vi "数据查询_数据查询.vi"() -> ()   [LabVIEW 2016]
uses:
  <vilib>/Utility/miscctls.llb/LVPointTypeDef.ctl
  <vilib>/Utility/miscctls.llb/LVRowAndColumnUnsignedTypeDef.ctl
  <vilib>/addons/database/_DB Variant To Data/Database Variant To Data.xnode
  SQL/database.lvlib
panel:
  out "连接的字符串":string
  out "选中数据表":string
  in  "查询":bool
  in  "结束日期":string="2020/01/01"
  in  "起始日期":string="2010/01/01"
  out "XY图":cluster{"data":timestamp[], "data":dbl[]}[](graph)
  in  "组合框":string(combo)
  out "数据表":string[][](table)
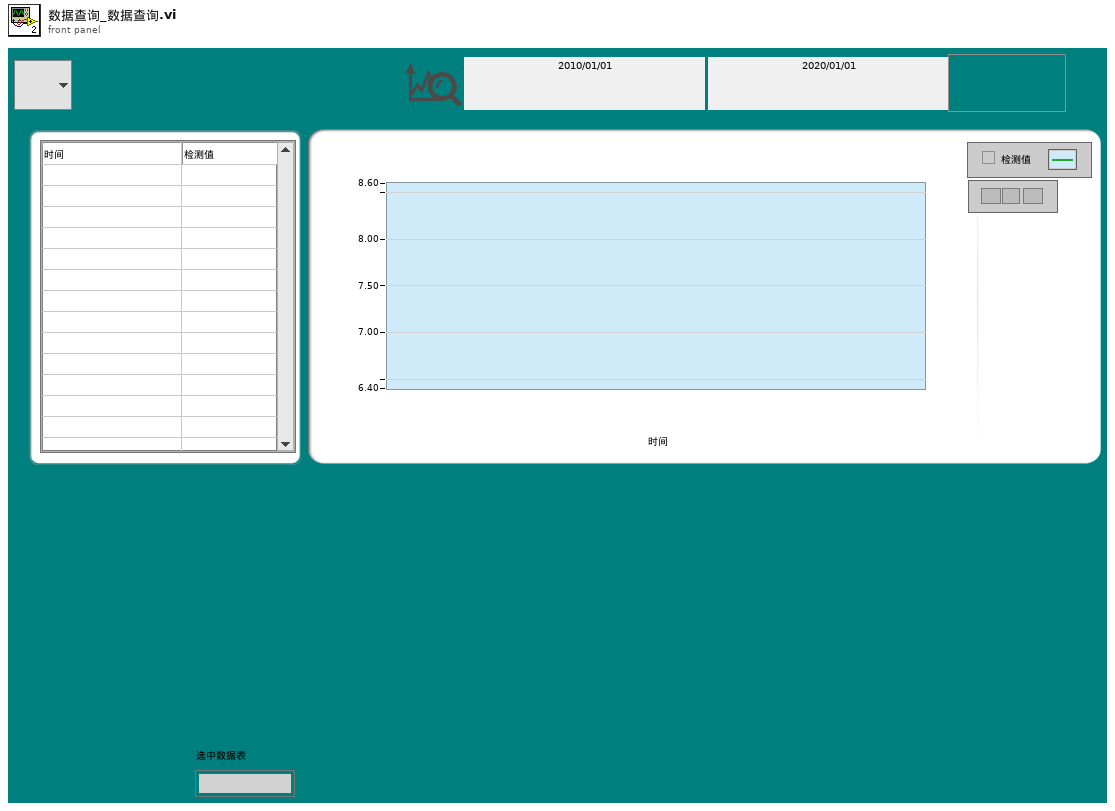
[diagram p1: front panel]
types:
  T1 = typedef "LVPointTypeDef.ctl" = cluster{"Horizontal":i16, "Vertical":i16}
  T2 = typedef "LVRowAndColumnUnsignedTypeDef.ctl" = cluster{"Row":u32, "Column":u32}
  T3 = typedef "LVPoint32TypeDef.ctl" = cluster{"Horizontal":i32, "Vertical":i32}
  T4 = typedef "LVPointDoubleTypeDef.ctl" = cluster{"Cursor X":dbl, "Cursor Y":dbl}
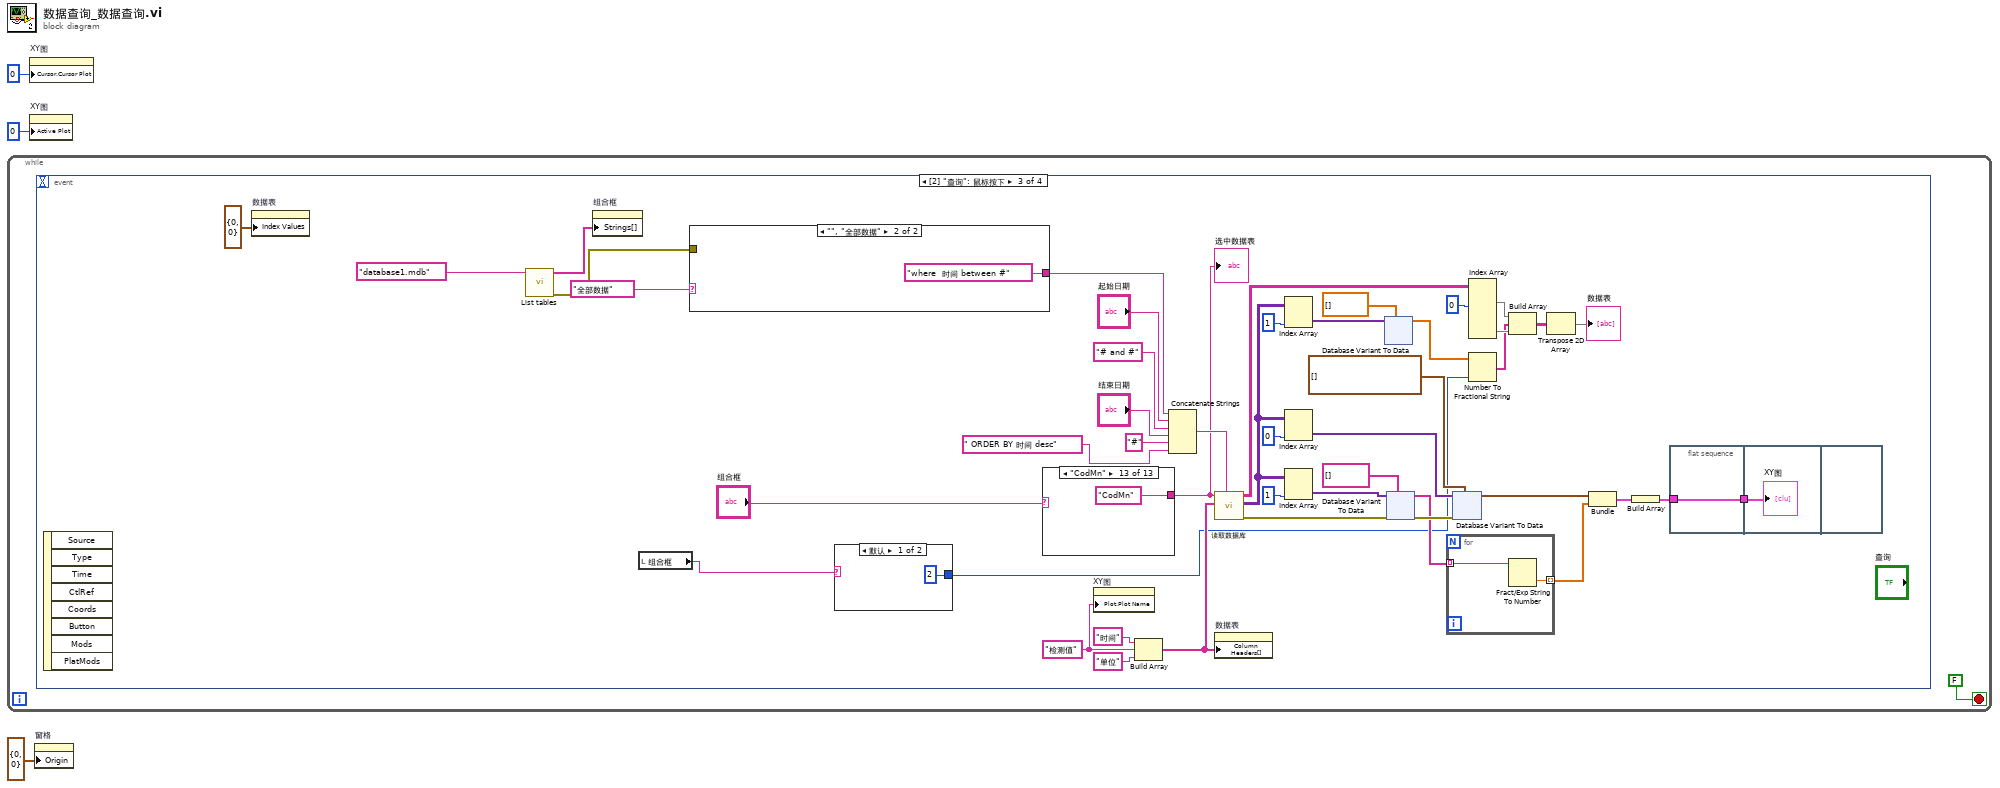
[diagram p0: block diagram]
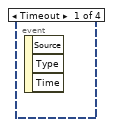
[diagram p2: hidden frame]
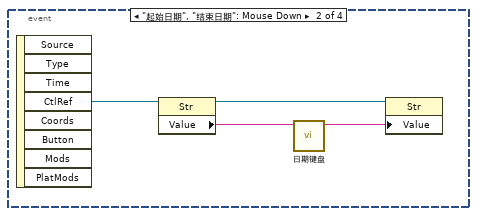
[diagram p3: hidden frame]
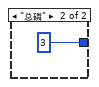
[diagram p4: hidden frame]
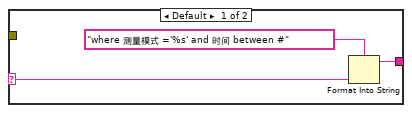
[diagram p5: hidden frame]
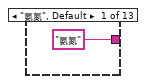
[diagram p6: hidden frame]
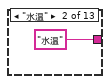
[diagram p7: hidden frame]
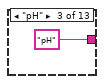
[diagram p8: hidden frame]
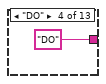
[diagram p9: hidden frame]
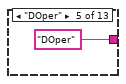
[diagram p10: hidden frame]
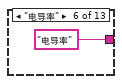
[diagram p11: hidden frame]
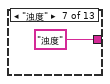
[diagram p12: hidden frame]
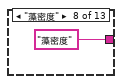
[diagram p13: hidden frame]
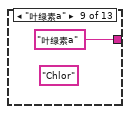
[diagram p14: hidden frame]
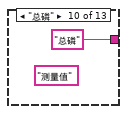
[diagram p15: hidden frame]
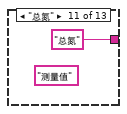
[diagram p16: hidden frame]
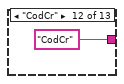
[diagram p17: hidden frame]
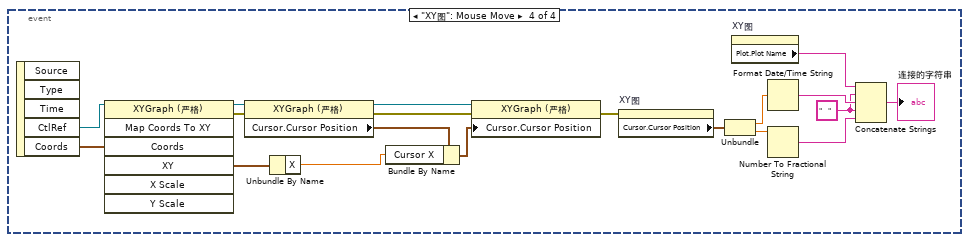
[diagram p18: hidden frame]
diagram:
  n1 = while {
    stop <- FALSE stop-if-true
    n2 = event shown="[2] \"查询\": 鼠标按下" {
      selector: _ -> [_ _ _ _]
      dyn-events: _ -> [_ _ _ _]
      timeout: _ -> [_ _ _ _]
      event Timeout {
        n3 = event-data() -> ()  [unwired: 1 in, 3 out]
      }
      event "起始日期", "结束日期": Mouse Down {
        n4 = event-data() -> ("CtlRef"=w8:refnum<vi>)  [unwired: 1 in, 7 out]
        n5 = property class="Str"(reference=w8) -> (reference out=w6:refnum<vi>, "Value"=w7:string)  [unwired: 1 in, 1 out]
        n6 = call "日期键盘.vi"("原值"=w7) -> ("x+y"=w5:string)  [unwired: 10 in]
        n7 = property class="Str"(reference=w6, "Value"=w5) -> ()  [unwired: 1 in, 2 out]
      }
      event "查询": Mouse Down {
        w26 = "检测值"
        n8 = event-data() -> ()  [unwired: 1 in, 8 out]
        n9 = property on="数据表" class="Tbl (严格)"("Index Values"=T2 {"Row"=0, "Column"=0} ("索引值")) -> ()  [unwired: 2 in, 2 out]
        n10 = call "List tables.vi"("database"="database1.mdb") -> ("error out"=w11:errorcluster, "tables"=w12:string[])  [unwired: 9 in]
        n11 = property on="组合框" class="CmbBox"("Strings[]"=w12) -> ()  [unwired: 2 in, 2 out]
        n12 = local read "组合框"() -> (w10:string)
        n13 = case shown="\"\", \"全部数据\"" "全部数据" ("工作模式") {
          selector: "全部数据" ("工作模式") -> [w59 _]
          tunnel: [w57 "where  时间 between #" ("condition")] -> w15
          tunnel: w11 -> [_ _]
          frame Default {
            n14 = Format Into String(format string="where 测量模式 ='%s' and 时间 between #" ("condition"), w59) -> (resulting string=w57:string)  [unwired: 2 in, 1 out]
          }
          frame "", "全部数据" {
          }
        }
        n15 = case shown="默认" w10 {
          tunnel: [i16 2 ("精度(6)") i16 3 ("精度(6)")] -> w9
          frame Default {
          }
          frame "总磷" {
          }
        }
        n16 = case shown="\"CodMn\"" "组合框" {
          tunnel: ["氨氮" "水温" "pH" "DO" "DOper" "电导率" "浊度" "藻密度" "叶绿素a" "总磷" "总氮" "CodCr" "CodMn"] -> w28
          frame "氨氮", Default {
          }
          frame "水温" {
          }
          frame "pH" {
          }
          frame "DO" {
          }
          frame "DOper" {
          }
          frame "电导率" {
          }
          frame "浊度" {
          }
          frame "藻密度" {
          }
          frame "叶绿素a" {
            (unwired) "Chlor"
          }
          frame "总磷" {
            (unwired) "测量值"
          }
          frame "总氮" {
            (unwired) "测量值"
          }
          frame "CodCr" {
          }
          frame "CodMn" {
          }
        }
        "选中数据表" <- w28
        n17 = property on="XY图" class="XYGraph (严格)"("Plot.Plot Name"=w26) -> ()  [unwired: 2 in, 2 out]
        n18 = Build Array("时间", w26, "单位" ("元素")) -> (w29:string[])
        n19 = Concatenate Strings(w15, "起始日期", "# and #" ("condition"), "结束日期", "#" ("condition"), " ORDER BY 时间 desc" ("字符串")) -> (w53:string)
        n20 = call "读取数据库.vi"("condition"=w53, "显示项"=w29, "组合框"=w28) -> ("error out"=w44:errorcluster, "data"=w23:variant[][], "表格"=w36:string[][])  [unwired: 5 in, 1 out]
        n21 = property on="数据表" class="Tbl (严格)"("Column Headers[]"=w29) -> ()  [unwired: 2 in, 2 out]
        n22 = Index Array(array=w23, index (col)=1 ("禁用的索引 (列)")) -> (element=w21:variant[])  [unwired: 1 in]
        n23 = Index Array(array=w23, index (col)=0 ("禁用的索引 (列)")) -> (element=w47:variant[])  [unwired: 1 in]
        n24 = Index Array(array=w23, index (col)=1 ("禁用的索引 (列)")) -> (element=w45:variant[])  [unwired: 1 in]
        n25 = xnode "Database Variant To Data"("database variant"=w21, "type"=sgl[] []) -> ("data"=w19:sgl[])  [unwired: 1 in, 1 out]
        n26 = xnode "Database Variant To Data"("database variant"=w45, "error in (no error)"=w44, "type"=string[] []) -> ("data"=w27:string[], "error out"=w43:errorcluster)
        n27 = for {
          tunnel: w27 -> [w100] mode=indexing
          tunnel: [w99] -> w14 mode=indexing
          n28 = Fract/Exp String To Number(string=w100) -> (number=w99:dbl)  [unwired: 3 in, 1 out]
        }
        n29 = xnode "Database Variant To Data"("database variant"=w47, "error in (no error)"=w43, "type"=timestamp[] []) -> ("data"=w38:timestamp[])  [unwired: 1 out]
        n30 = Index Array(array=w36, index (col) #1=0 ("禁用的索引 (列)")) -> (element #1=w34:string[], element #3=w24:string[])  [unwired: 5 in, 1 out]
        n31 = Number To Fractional String(number=w19, precision (6)=w9) -> (F-format string=w18:string[])  [unwired: 2 in]
        n32 = Build Array(w34, w18, w24) -> (w33:string[][])
        n33 = Transpose 2D Array(2D array=w33) -> (transposed array=→"数据表":string[][])
        n34 = Bundle("data"=w38, w14) -> (w39:cluster{"data":timestamp[], dbl[]})  [unwired: 1 in]
        n35 = Build Array(w39) -> (w40:cluster{"data":timestamp[], dbl[]}[])
        n36 = flat-sequence {
          tunnel: [w114] -> w41
          tunnel: w40 -> [w114]
          tunnel: w41 -> [w115]
          frame #0 {
          }
          frame #1 {
            "XY图" <- w115
          }
          frame #2 {
          }
        }
      }
      event "XY图": Mouse Move {
        w217 = "   " ("字符串")
        n37 = event-data() -> ("CtlRef"=w224:refnum<vi>, "Coords"=w223:T3)  [unwired: 1 in, 3 out]
        n38 = invoke class="XYGraph (严格)" method="Map Coords To XY"(reference=w224, "Coords"=w223) -> (reference out=w212:refnum<vi>, error out=w210:errorcluster, "XY"=w213:cluster{"X":dbl, "Y":dbl})  [unwired: 5 in, 4 out]
        n39 = property class="XYGraph (严格)"(reference=w212, error in=w210) -> (reference out=w211:refnum<vi>, error out=w209:errorcluster, "Cursor.Cursor Position"=w208:T4)
        n40 = Unbundle By Name(w213) -> ("X"=w207:dbl)
        n41 = Bundle By Name(cluster=w208, "Cursor X"=w207) -> (w206:T4)
        n42 = property class="XYGraph (严格)"(reference=w211, error in=w209, "Cursor.Cursor Position"=w206) -> (error out=w222:errorcluster)  [unwired: 1 out]
        n43 = property on="XY图" class="XYGraph (严格)"(error in=w222) -> ("Cursor.Cursor Position"=w220:T4)  [unwired: 1 in, 2 out]
        n44 = Unbundle(w220) -> ("Cursor X"=w219:dbl, "Cursor Y"=w216:dbl)
        n45 = property on="XY图" class="XYGraph (严格)"() -> ("Plot.Plot Name"=w214:string)  [unwired: 2 in, 2 out]
        n46 = Format Date/Time String(seconds (now)=w219) -> (date/time string=w218:string)  [unwired: 2 in]
        n47 = Number To Fractional String(number=w216) -> (F-format string=w215:string)  [unwired: 3 in]
        n48 = Concatenate Strings(w214, w217, w218, w217, w215) -> (→"连接的字符串":string)
      }
    }
  }
  n49 = property on="XY图" class="XYGraph (严格)"("Cursor.Cursor Plot"=0 ("游标.游标关联曲线")) -> ()  [unwired: 2 in, 2 out]
  n50 = property on="XY图" class="XYGraph (严格)"("Active Plot"=u32 0 ("活动曲线")) -> ()  [unwired: 2 in, 2 out]
  n51 = property on="窗格" class="Pane"("Origin"=T1 {"Horizontal"=0, "Vertical"=0} ("原点")) -> ()  [unwired: 2 in, 2 out]
